vi "ArrayTransformations.vi"(1 "Input":sgl[][](array[numeric]) format="%#_13g", 2 "Option":string(combo)) -> (0 "Output":sgl[][](array[numeric]) format="%#_13g")   [LabVIEW 2014]
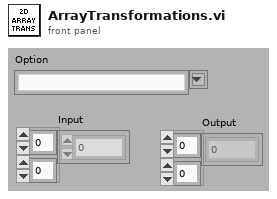
[diagram p1: front panel]
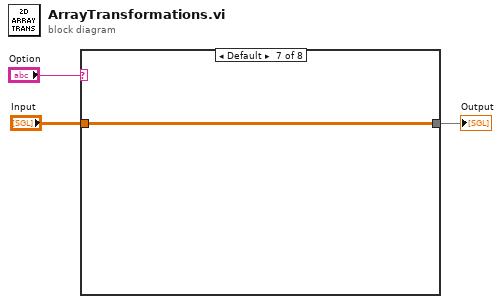
[diagram p0: block diagram]
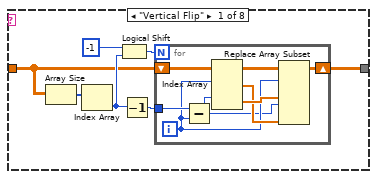
[diagram p2: hidden frame]
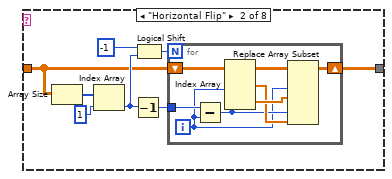
[diagram p3: hidden frame]
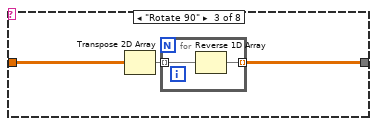
[diagram p4: hidden frame]
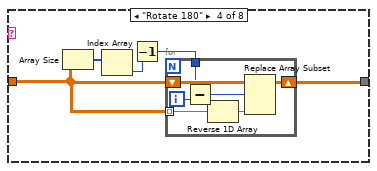
[diagram p5: hidden frame]
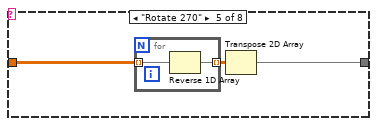
[diagram p6: hidden frame]
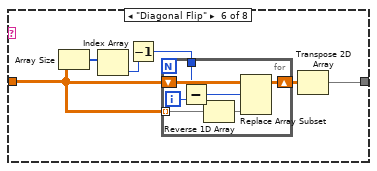
[diagram p7: hidden frame]
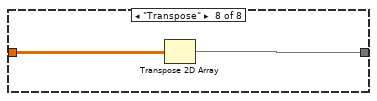
[diagram p8: hidden frame]
diagram:
  n1 = case shown="Default" "Option" {
    tunnel: "Input" -> [w5 w19 w34 w39 w51 w56 w68 w70]
    tunnel: [w4 w18 w33 w38 w50 w55 w68 w69] -> w1
    frame "Vertical Flip" {
      n2 = Array Size(array=w5) -> (size(s)=w10:i32[])
      n3 = Index Array(array=w10) -> (element=w8:i32)  [unwired: 1 in]
      n4 = Logical Shift(y=i8 -1, x=w8) -> (x << y=w9:i32)
      n5 = Decrement(x=w8) -> (x-1=w6:i32)
      n6 = for {
        N: w9 -> [_]
        shift-right: [w17] -> w4
        shift-left: w5 -> [w16]
        tunnel: w6 -> [w13]
        i -> [w12]
        n7 = Subtract(x=w13, y=w12) -> (x-y=w11:i32)
        n8 = Index Array(array=w16, index (row) #1=w12, index (row) #2=w11) -> (element #1=w14:sgl[], element #2=w15:sgl[])  [unwired: 2 in]
        n9 = Replace Array Subset(array=w16, new element #1=w15, index (row) #1=w12, new element #2=w14, index (row) #2=w11) -> (w17:sgl[][])  [unwired: 2 in]
      }
    }
    frame "Horizontal Flip" {
      n10 = Array Size(array=w19) -> (size(s)=w21:i32[])
      n11 = Index Array(array=w21, index=1) -> (element=w23:i32)
      n12 = Decrement(x=w23) -> (x-1=w25:i32)
      n13 = Logical Shift(y=i8 -1, x=w23) -> (x << y=w22:i32)
      n14 = for {
        N: w22 -> [_]
        shift-right: [w32] -> w18
        shift-left: w19 -> [w31]
        tunnel: w25 -> [w28]
        i -> [w26]
        n15 = Subtract(x=w28, y=w26) -> (x-y=w27:i32)
        n16 = Index Array(array=w31, index (col) #1=w26, index (col) #2=w27) -> (element #1=w29:sgl[], element #2=w30:sgl[])  [unwired: 2 in]
        n17 = Replace Array Subset(array=w31, new element #1=w30, index (col) #1=w26, new element #2=w29, index (col) #2=w27) -> (w32:sgl[][])  [unwired: 2 in]
      }
    }
    frame "Rotate 90" {
      n18 = Transpose 2D Array(2D array=w34) -> (transposed array=w35:sgl[][])
      n19 = for {
        tunnel: w35 -> [w37] mode=indexing
        tunnel: [w36] -> w33 mode=indexing
        n20 = Reverse 1D Array(array=w37) -> (reversed array=w36:sgl[])
      }
    }
    frame "Rotate 180" {
      n21 = Array Size(array=w39) -> (size(s)=w42:i32[])
      n22 = Index Array(array=w42) -> (element=w40:i32)  [unwired: 1 in]
      n23 = Decrement(x=w40) -> (x-1=w41:i32)
      n24 = for {
        shift-right: [w49] -> w38
        shift-left: w39 -> [w48]
        tunnel: w41 -> [w46]
        tunnel: w39 -> [w43] mode=indexing
        i -> [w47]
        n25 = Subtract(x=w46, y=w47) -> (x-y=w45:i32)
        n26 = Reverse 1D Array(array=w43) -> (reversed array=w44:sgl[])
        n27 = Replace Array Subset(array=w48, new element=w44, index (row)=w45) -> (w49:sgl[][])  [unwired: 1 in]
      }
    }
    frame "Rotate 270" {
      n28 = for {
        tunnel: w51 -> [w54] mode=indexing
        tunnel: [w53] -> w52 mode=indexing
        n29 = Reverse 1D Array(array=w54) -> (reversed array=w53:sgl[])
      }
      n30 = Transpose 2D Array(2D array=w52) -> (transposed array=w50:sgl[][])
    }
    frame "Diagonal Flip" {
      n31 = Array Size(array=w56) -> (size(s)=w58:i32[])
      n32 = Index Array(array=w58) -> (element=w60:i32)  [unwired: 1 in]
      n33 = Decrement(x=w60) -> (x-1=w59:i32)
      n34 = for {
        shift-right: [w67] -> w57
        shift-left: w56 -> [w66]
        tunnel: w59 -> [w64]
        tunnel: w56 -> [w61] mode=indexing
        i -> [w65]
        n35 = Subtract(x=w64, y=w65) -> (x-y=w63:i32)
        n36 = Reverse 1D Array(array=w61) -> (reversed array=w62:sgl[])
        n37 = Replace Array Subset(array=w66, new element=w62, index (row)=w63) -> (w67:sgl[][])  [unwired: 1 in]
      }
      n38 = Transpose 2D Array(2D array=w57) -> (transposed array=w55:sgl[][])
    }
    frame Default {
    }
    frame "Transpose" {
      n39 = Transpose 2D Array(2D array=w70) -> (transposed array=w69:sgl[][])
    }
  }
  "Output" <- w1
